vi "Tracepoint_OpenFiles.vi"(8 "error in (no error)":errorcluster, 9 "max open files":i32, 10 "open files":i32, 11 "Qbus":refnum<class "Qbus.lvclass">) -> (0 "error out":errorcluster)   [LabVIEW 2017, in "CmsDataEventCreator.lvlib"]
uses:
  <vilib>/addons/InsightCM/Devices/Shared/Cms/CmsDataEventCreator/CmsDataEventCreator.lvlib
  <vilib>/addons/Qbus/Qbus.lvclass
  <vilib>/addons/TraceLogger/TraceLogger.lvlib
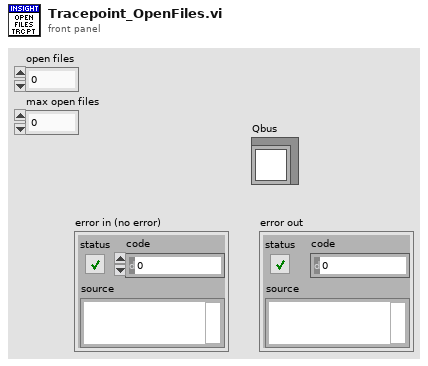
[diagram p1: front panel]
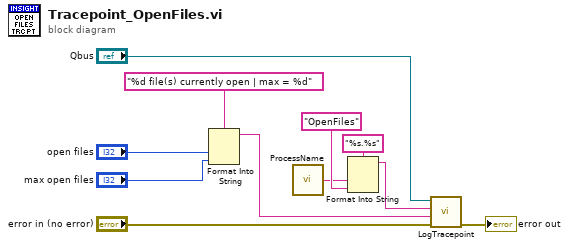
[diagram p0: block diagram]
diagram:
  n1 = Format Into String(format string="%d file(s) currently open | max = %d", "open files", "max open files") -> (resulting string=w4:string)  [unwired: 2 in, 1 out]
  n2 = call <vilib>:"ProcessName.vi"() -> ("process name"=w5:string)  [unwired: 5 in]
  n3 = Format Into String(format string="%s.%s", w5, "OpenFiles" ("tracepoint")) -> (resulting string=w7:string)  [unwired: 2 in, 1 out]
  n4 = call <vilib>:"LogTracepoint.vi"("error in (no error)"="error in (no error)", "log string"=w4, "tracepoint"=w7, "qbus in"="Qbus") -> ("error out"=→"error out":errorcluster)  [unwired: 6 in, 1 out]
